vi "Write LogPath.vi"(8 "error in (no error)":errorcluster, 10 "LogPath":path, 11 "Logs in":refnum<class "Logs.lvclass">) -> (0 "error out":errorcluster, 3 "Logs out":refnum<class "Logs.lvclass">)   [LabVIEW 2019, in "Logs.lvclass"]
uses:
  Logs.lvclass
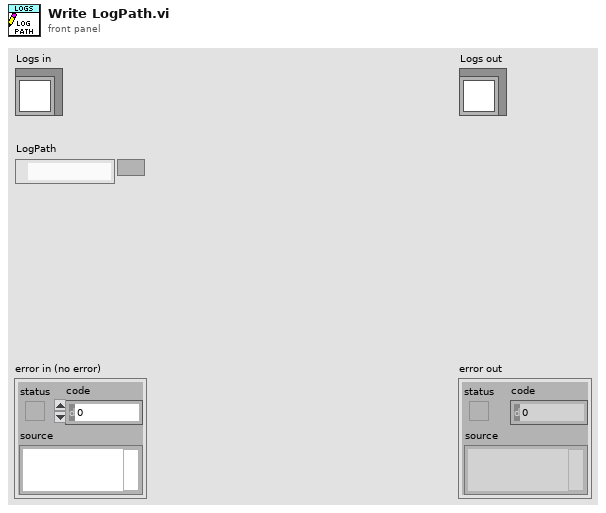
[diagram p1: front panel]
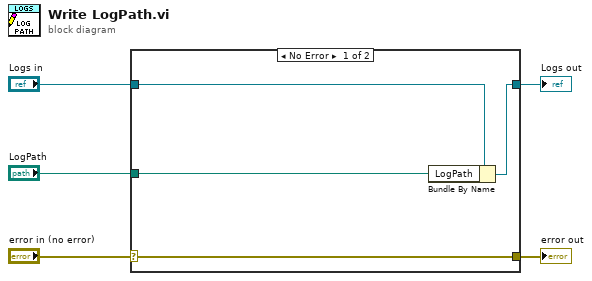
[diagram p0: block diagram]
diagram:
  n1 = case shown="No Error" "error in (no error)" {
    selector: "error in (no error)" -> [w9 w10]
    tunnel: [w9 w10] -> w4
    tunnel: [w7 w11] -> w2
    tunnel: "Logs in" -> [w8 w11]
    tunnel: "LogPath" -> [w6 _]
    frame No Error {
      n2 = Bundle By Name(cluster=w8, "LogPath"=w6) -> (w7:refnum<class "Logs.lvclass">)
    }
    frame Error {
    }
  }
  "error out" <- w4
  "Logs out" <- w2
